vi "18.6 Color Threshold.vi"() -> ()   [LabVIEW 2017]
doc: "This example shows the advantages of using the HSL color space over the RGB color space to perform color inspection in certain situations."
uses:
  <vilib>/vision/NI_Vision_Development_Module.lvlib
panel:
  in  "Stop":bool
  in  "Test Image":enum32{"Image 1", "Image 2"}(radio)
  in  "Threshold Color Mode":enum32{"RGB", "HSL"}(radio)=enum."HSL"
  in  "Blue or Luminance":cluster{i32, i32}(slide)={20, 217} scale=0.0..255.0
  in  "Green or Saturation":cluster{i32, i32}(slide)={20, 233} scale=0.0..255.0
  in  "Red or Hue":cluster{i32, i32}(slide)={42, 99} scale=0.0..255.0
  out "Original Image":T1(plugin-control)
  out "Threshold Image":T1(plugin-control)
  # "Minimum"
  # "Maximum"
  # "Minimum"
  # "Maximum"
  # "Minimum"
  # "Maximum"
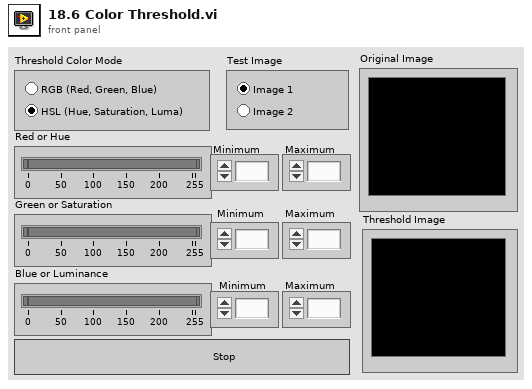
[diagram p1: front panel]
types:
  T1 = typedef "IMAQ Image.ctl" = refnum<image>
  T2 = typedef "Image Type" = u32
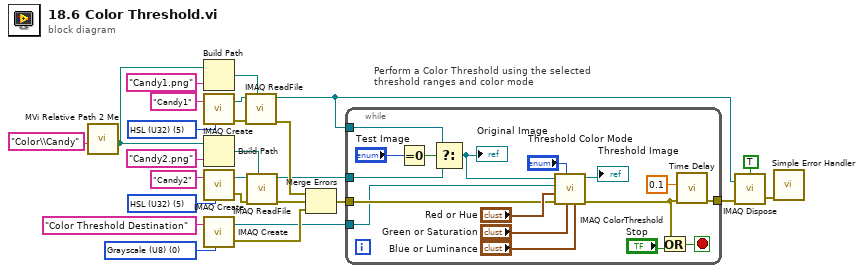
[diagram p0: block diagram]
diagram:
  w8 = T2 5 items=["Grayscale (U8)", "Grayscale (I16)", "Grayscale (SGL)", "Complex (CSG)", "RGB (U32)", "HSL (U32)", "RGB (U64)", "Grayscale (U16)"] ("Image Type")
  w9 = T2 0 items=["Grayscale (U8)", "Grayscale (I16)", "Grayscale (SGL)", "Complex (CSG)", "RGB (U32)", "HSL (U32)", "RGB (U64)", "Grayscale (U16)"] ("Image Type")
  w10 = T2 5 items=["Grayscale (U8)", "Grayscale (I16)", "Grayscale (SGL)", "Complex (CSG)", "RGB (U32)", "HSL (U32)", "RGB (U64)", "Grayscale (U16)"] ("Image Type")
  # "Perform a Color Threshold using the selected threshold ranges and color mode"
  n1 = call "MVi Relative Path 2 Me.vi"("Relative Path"="Color\\Candy") -> ("Appended Dir"=w7:path)  [unwired: 5 in, 1 out]
  n2 = Build Path(base path=w7, name or relative path="Candy1.png") -> (appended path=w22:path)
  n3 = call "IMAQ Create"("Image Name"="Candy1", "Image Type"=w8) -> ("New Image"=w21:T1, "error out"=w20:errorcluster)  [unwired: 3 in]
  n4 = Build Path(base path=w7, name or relative path="Candy2.png") -> (appended path=w16:path)
  n5 = call "IMAQ Create"("Image Name"="Candy2", "Image Type"=w10) -> ("New Image"=w19:T1, "error out"=w18:errorcluster)  [unwired: 3 in]
  n6 = call "IMAQ Create"("Image Name"="Color Threshold Destination", "Image Type"=w9) -> ("New Image"=w4:T1, "error out"=w12:errorcluster)  [unwired: 3 in]
  n7 = call "IMAQ ReadFile"("File Path"=w22, "error in (no error)"=w20, "Image"=w21) -> ("error out"=w13:errorcluster, "Image Out"=w5:T1)  [unwired: 4 in, 3 out]
  n8 = call "IMAQ ReadFile"("File Path"=w16, "error in (no error)"=w18, "Image"=w19) -> ("error out"=w14:errorcluster, "Image Out"=w3:T1)  [unwired: 4 in, 3 out]
  n9 = Merge Errors(w13, w14, w12) -> (w11:errorcluster)
  n10 = while {
    tunnel: w4 -> [w27]
    tunnel: w5 -> [w39]
    tunnel: w3 -> [w38]
    tunnel: [w29] -> w15
    tunnel: w11 -> [w30]
    stop <- w35 stop-if-true
    n11 = Equal To 0?(x="Test Image") -> (x = 0?=w40:bool)
    n12 = Select(t=w39, s=w40, f=w38) -> (s? t:f=w34:T1)
    "Original Image" <- w34
    n13 = call "IMAQ ColorThreshold"("Blue or Luma or Val or Inten Range"="Blue or Luminance", "Green or Sat Range"="Green or Saturation", "Color Mode"="Threshold Color Mode", "error in (no error)"=w30, "Red or Hue Range"="Red or Hue", "Image Dst"=w27, "Image Src"=w34) -> ("error out"=w32:errorcluster, "Image Dst Out"=→"Threshold Image":T1)  [unwired: 3 in]
    n14 = Or(x=w32, y="Stop") -> (x .or. y?=w35:bool)
    n15 = call "Time Delay"("error in (no error)"=w32, "Delay Time (s)"=0.1) -> ("error out"=w29:errorcluster)  [unwired: 9 in]
  }
  n16 = call "IMAQ Dispose"("All Images? (No)"=TRUE, "Image"=w5, "error in (no error)"=w15) -> ("error out"=w2:errorcluster)  [unwired: 3 in]
  n17 = call <vilib>:"Simple Error Handler.vi"("error in (no error)"=w2) -> ()  [unwired: 4 in, 5 out]
